vi "timeout.vi"(8 "error in (no error)":errorcluster, 11 "seconds to wait":dbl=0.2 min=0.2) -> (0 "error IO":errorcluster)   [LabVIEW 2017]
panel:
  in  "stop":bool
  out "Slide":u8(slide) caption="Таймаут" scale=0.0..100.0
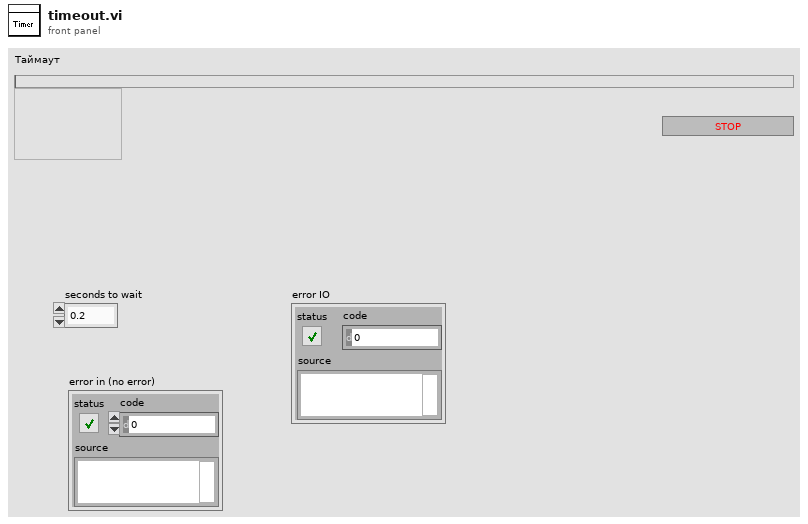
[diagram p1: front panel]
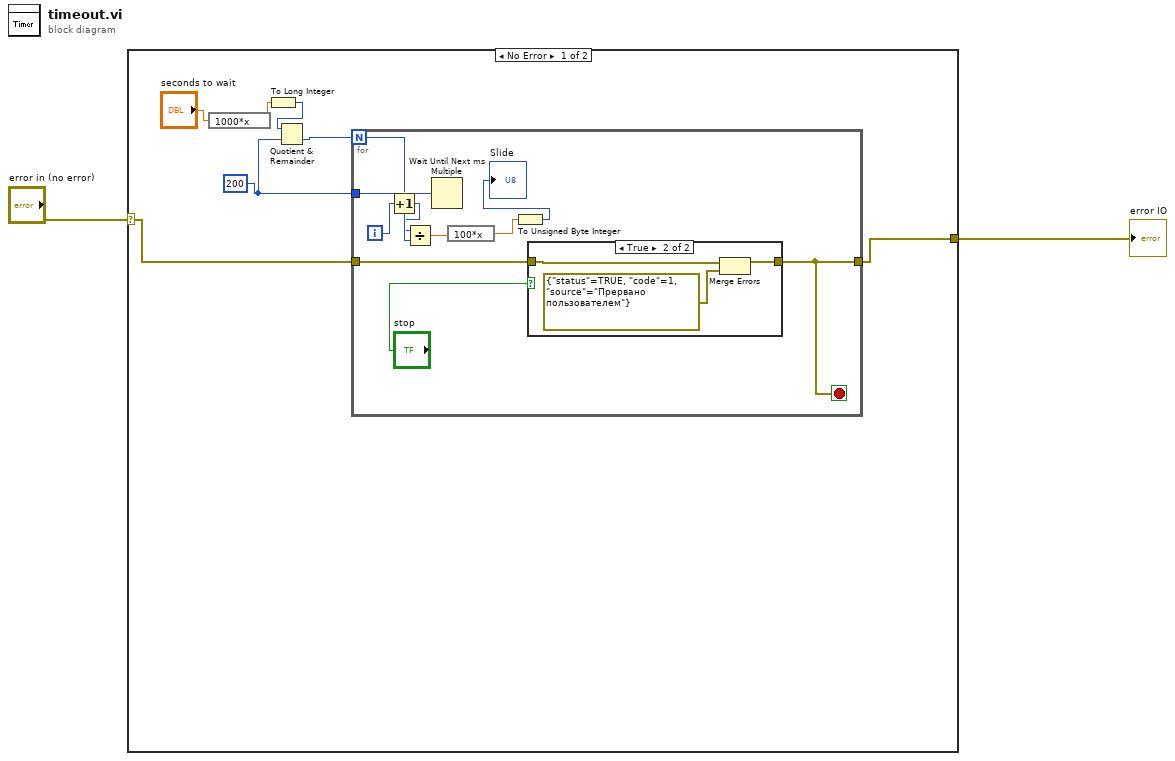
[diagram p0: block diagram]
diagram:
  n1 = case shown="No Error" "error in (no error)" {
    selector: "error in (no error)" -> [w4 w24]
    tunnel: [w3 w24] -> w1
    frame No Error {
      w6 = 200 ("millisecond multiple")
      n2 = expression code="1000*x"("seconds to wait") -> (w8:dbl)
      n3 = To Long Integer(number=w8) -> (32bit integer=w7:i32)
      n4 = Quotient & Remainder(x=w7, y=w6) -> (floor(x/y)=w5:i32)  [unwired: 1 out]
      n5 = for {
        N: w5 -> [w18]
        tunnel: w6 -> [w19]
        tunnel: w4 -> [w11]
        tunnel: [w10] -> w3
        i -> [w14]
        stop <- w10 stop-if-true
        n6 = Increment(x=w14) -> (x+1=w13:i32)
        n7 = Divide(x=w13, y=w18) -> (x/y=w17:dbl)
        n8 = Wait Until Next ms Multiple(millisecond multiple=w19) -> ()  [unwired: 1 out]
        n9 = expression code="100*x"(w17) -> (w16:dbl)
        n10 = To Unsigned Byte Integer(number=w16) -> (unsigned 8bit integer=→"Slide":u8)
        n11 = case shown="True" "stop" {
          tunnel: w11 -> [w20 w22]
          tunnel: [w20 w23] -> w10
          frame False {
          }
          frame True {
            n12 = Merge Errors(w22, errorcluster {"status"=TRUE, "code"=1, "source"="Прервано пользователем"} ("error constant")) -> (w23:errorcluster)
          }
        }
      }
    }
    frame Error {
    }
  }
  "error IO" <- w1
